vi "Relee.vi"() -> ()   [LabVIEW 2018]
uses:
  <vilib>/MakerHub/LINX/Public/Peripherals/Digital/Digital Write 1 Chan.vi
  <vilib>/MakerHub/LINX/Public/Peripherals/Digital/Digital Write N Chans.vi
  <vilib>/MakerHub/LINX/Private/Local IO/LinxDigitalWrite.vi
  <vilib>/MakerHub/LINX/Public/Utilities/Check Channel.vi
  <vilib>/MakerHub/LINX/Public/Utilities/Open Serial.vi
  <vilib>/MakerHub/LINX/Private/Utilties/Generate Error.vi
  <vilib>/MakerHub/LINX/LMH-LINX.lvlib
panel:
  in  "Releu Nr.2":bool
  in  "Releu Nr.8":bool
  in  "Releu Nr.7":bool
  in  "Releu Nr.6":bool
  in  "Releu Nr.5":bool
  in  "Releu Nr.4":bool
  in  "Releu Nr.3":bool
  in  "Releu Nr.1":bool
  in  "?":bool
  in  "Serial Port":refnum<visa-resource-name>="N/A"
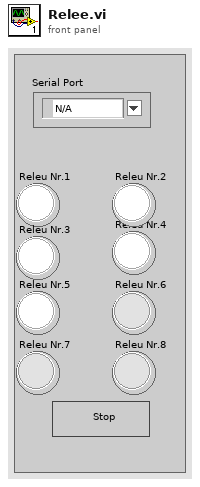
[diagram p1: front panel]
types:
  T1 = typedef "LMH-LINX.lvlib/LINX Ref.ctl" = cluster{"IO":T2, "Interface":T3, "LINX Device Config":T4}
  T2 = typedef "LMH-LINX.lvlib/Platform.ctl" = enum16{"Remote", "Local"}
  T3 = typedef "LMH-LINX.lvlib/Interface.ctl" = enum16{"Serial", "TCP"}
  T4 = typedef "LMH-LINX.lvlib/Device.lvlib/LINX Device Config.ctl" = cluster{"Interface":T3, "COM Port":refnum<visa-resource-name>, "TCP Configuration":T5, "Device Family":u8, "Device ID":u8, "Device Name":string, "TCP Ref":refnum<k5>, "Channels":T6}
  T5 = typedef "LMH-LINX.lvlib/Device.lvlib/TCP Config.ctl" = cluster{"IP Address":string, "Port":u16}
  T6 = typedef "LMH-LINX.lvlib/Channels.ctl" = cluster{"DI":u8[], "DO":u8[], "AI":u8[], "AO":u8[], "PWM":u8[], "QE":u8[], "UART":u8[], "I2C 2":u8[], "SPI":u8[], "CAN":u8[], "Servo":u8[], "AI Ref (V)":dbl, "AI Resolution (Bits)":u8, "AO Ref (V)":dbl, "AO Resolution (Bits)":u8}
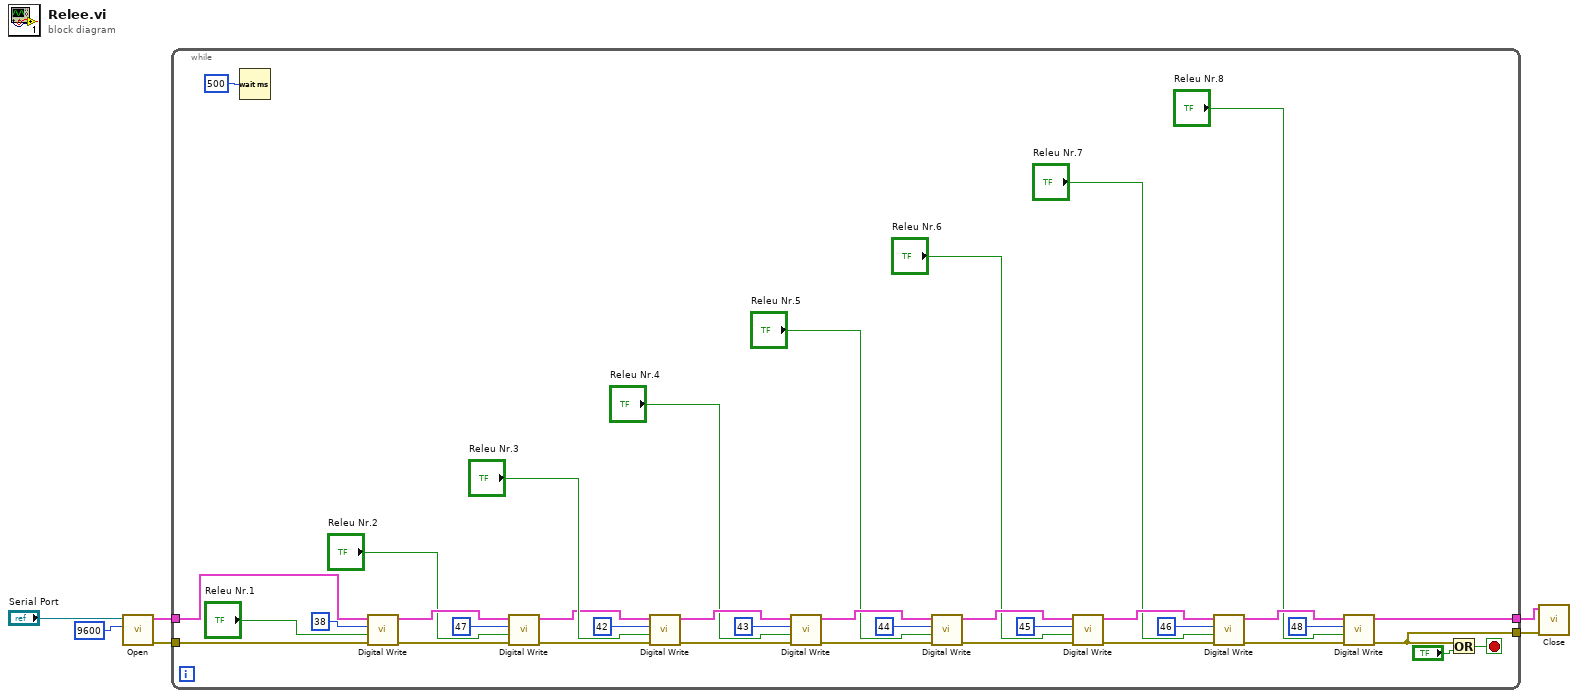
[diagram p0: block diagram]
diagram:
  n1 = call-poly <vilib>:"Open.vi"("Baud Rate Override"=u32 9600, "Serial Port"="Serial Port") -> ("Error Out"=w5:errorcluster, "LINX Resource"=w6:T1)  [unwired: 7 in, 1 out]
  n2 = while {
    tunnel: w6 -> [w41]
    tunnel: w5 -> [w42]
    tunnel: [w38] -> w4
    tunnel: [w35] -> w3
    stop <- w37 stop-if-true
    n3 = Wait (ms)(milliseconds to wait=u32 500) -> ()  [unwired: 1 out]
    n4 = call-poly <vilib>:"Digital Write.vi"("Error In"=w42, "Output Value"="Releu Nr.1", "DO Channel"=u8 38, "LINX Resource"=w41) -> ("Error Out"=w9:errorcluster, "LINX Resource"=w10:T1)  [unwired: 6 in]
    n5 = call-poly <vilib>:"Digital Write.vi"("Error In"=w9, "Output Value"="Releu Nr.2", "DO Channel"=u8 47, "LINX Resource"=w10) -> ("Error Out"=w12:errorcluster, "LINX Resource"=w11:T1)  [unwired: 6 in]
    n6 = call-poly <vilib>:"Digital Write.vi"("Error In"=w12, "Output Value"="Releu Nr.3", "DO Channel"=u8 42, "LINX Resource"=w11) -> ("Error Out"=w33:errorcluster, "LINX Resource"=w34:T1)  [unwired: 6 in]
    n7 = call-poly <vilib>:"Digital Write.vi"("Error In"=w33, "Output Value"="Releu Nr.4", "DO Channel"=u8 43, "LINX Resource"=w34) -> ("Error Out"=w31:errorcluster, "LINX Resource"=w32:T1)  [unwired: 6 in]
    n8 = call-poly <vilib>:"Digital Write.vi"("Error In"=w31, "Output Value"="Releu Nr.5", "DO Channel"=u8 44, "LINX Resource"=w32) -> ("Error Out"=w29:errorcluster, "LINX Resource"=w30:T1)  [unwired: 6 in]
    n9 = call-poly <vilib>:"Digital Write.vi"("Error In"=w29, "Output Value"="Releu Nr.6", "DO Channel"=u8 45, "LINX Resource"=w30) -> ("Error Out"=w27:errorcluster, "LINX Resource"=w28:T1)  [unwired: 6 in]
    n10 = call-poly <vilib>:"Digital Write.vi"("Error In"=w27, "Output Value"="Releu Nr.7", "DO Channel"=u8 46, "LINX Resource"=w28) -> ("Error Out"=w25:errorcluster, "LINX Resource"=w26:T1)  [unwired: 6 in]
    n11 = call-poly <vilib>:"Digital Write.vi"("Error In"=w25, "Output Value"="Releu Nr.8", "DO Channel"=u8 48, "LINX Resource"=w26) -> ("Error Out"=w35:errorcluster, "LINX Resource"=w38:T1)  [unwired: 6 in]
    n12 = Or(x=w35, y="?") -> (x .or. y?=w37:bool)
  }
  n13 = call <vilib>:"Close.vi"("Error In"=w3, "LINX Resource"=w4) -> ()  [unwired: 9 in, 1 out]
